vi "Config_Param_Emballage.vi"(0 "Choix imprimante":T1(ring), 5 "Dec.Droite":string="^LH70,20", 11 "error in (no error)":errorcluster caption="entrée d'erreur (pas d'erreur)") -> (4 "Output VISA Imprimante":refnum<visa-resource-name>="none", 6 "New_Dec.Droite":string="^LH70,20", 15 "error out":errorcluster caption="sortie d'erreur")   [LabVIEW 2020]
panel:
  in  "OK":bool
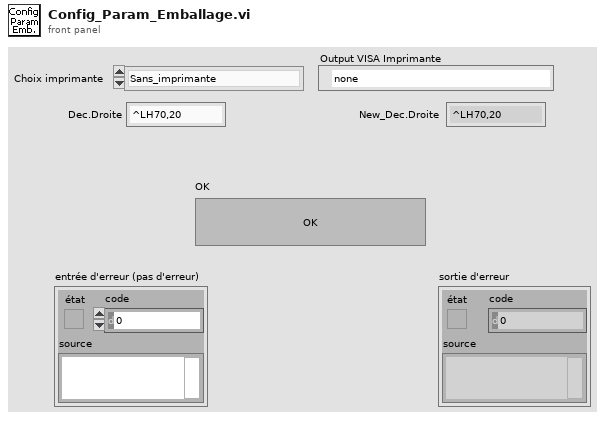
[diagram p1: front panel]
types:
  T1 = enum16{"Sans_imprimante", "Zebra_Medic_emballage2", "Zebra_Medic_2", "Zebra_Medic_1", "Zebra_Flat_emballage"}
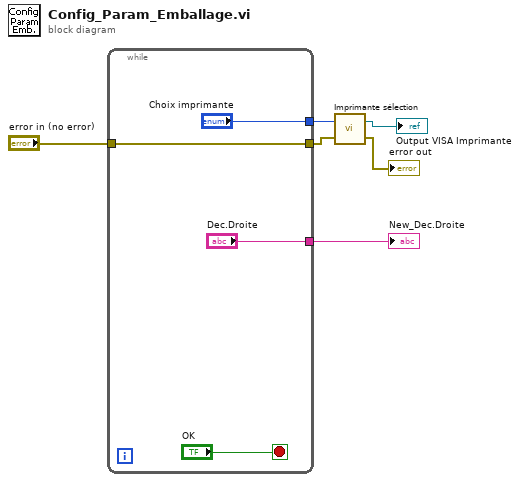
[diagram p0: block diagram]
diagram:
  n1 = while {
    tunnel: ["Dec.Droite"] -> w6
    tunnel: ["Choix imprimante"] -> w5
    tunnel: [w7] -> w2
    tunnel: "error in (no error)" -> [w7]
    stop <- "OK" stop-if-true
  }
  "New_Dec.Droite" <- w6
  n2 = call "Imprimante sélection.vi"("entrée d'erreur"=w2, "Choix imprimante"=w5) -> ("sortie d'erreur"=→"error out":errorcluster, "Output ressource VISA"=→"Output VISA Imprimante":refnum<visa-resource-name>)
